vi "Fetch Waveforms for One Record.vi"(8 "error in (no error)":errorcluster, 9 "min record length":i32[](array[numeric]), 10 "fetch record number":i32, 11 "connections":T1[](array[typedef])) -> (0 "error out":errorcluster, 1 "waveforms":waveform(dbl)[](array[waveform]), 2 "sites":i32[](array[numeric]), 3 "pins or relay names":string[](array[string]))   [LabVIEW 2021, in "PMIC Common.lvlib"]
uses:
  PMIC Common.lvlib
  <instrlib>/niScope/Controls/niScope timestamp type.ctl
  <instrlib>/niScope/Acquire/Fetch/niScope Multi Fetch WDT.vi
  <vilib>/Plug-In SDKs/Clients/Session Management V1/Session Reservation/Connection.ctl
  <vilib>/Plug-In SDKs/Clients/Session Management V1/Session Reservation/Session Reservation.lvclass
  <vilib>/Plug-In SDKs/Sessions/niScope/Connection with Session.ctl
  <vilib>/Plug-In SDKs/Sessions/niScope/NI Session Management niScope.lvlib
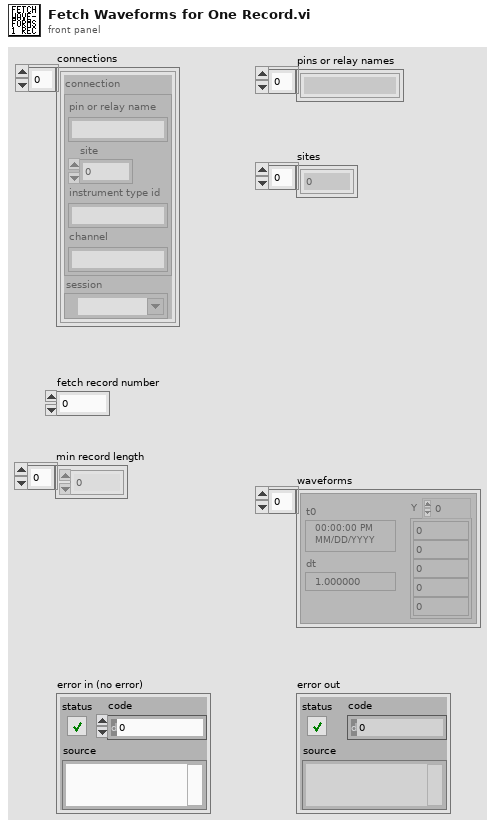
[diagram p1: front panel]
types:
  T1 = typedef "NI Session Management niScope.lvlib/Connection with Session.ctl" = cluster{"connection":T2, "session":refnum<k15>}
  T2 = typedef "NI Session Management V1 Client.lvlib/Session Reservation.lvclass/Connection.ctl" = cluster{"pin or relay name":string, "site":i32, "instrument type id":string, "channel":string}
  T3 = typedef "niScope timestamp type.ctl" = i32
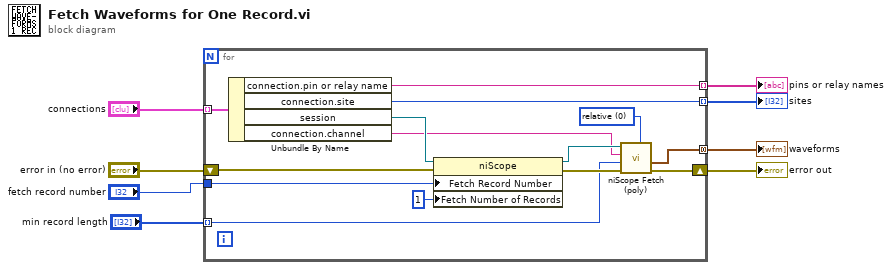
[diagram p0: block diagram]
diagram:
  n1 = for {
    tunnel: "connections" -> [w22] mode=indexing
    tunnel: "fetch record number" -> [w20]
    shift-right: [w14] -> w1
    shift-left: "error in (no error)" -> [w21]
    tunnel: [w13] -> w2 mode=concatenating
    tunnel: "min record length" -> [w12] mode=indexing
    tunnel: [w11] -> w3 mode=indexing
    tunnel: [w10] -> w4 mode=indexing
    w9 = T3 0 items=["relative", "absolute"] ("timestamp Type")
    n2 = Unbundle By Name(w22) -> ("connection.pin or relay name"=w11:string, "connection.site"=w10:i32, "session"=w16:refnum<k15>, "connection.channel"=w15:string)
    n3 = property class="niScope"(reference=w16, error in=w21, "Fetch Record Number"=w20, "Fetch Number of Records"=1 ("Fetch:Fetch Number of Records")) -> (reference out=w17:refnum<k15>, error out=w18:errorcluster)
    n4 = call-poly <instrlib>:"niScope Fetch (poly).vi"("timestamp Type"=w9, "error in"=w18, "numSamples"=w12, "channels"=w15, "instrument handle"=w17) -> ("error out"=w14:errorcluster, "wfm"=w13:waveform(dbl)[])  [unwired: 3 in, 2 out]
  }
  "sites" <- w4
  "pins or relay names" <- w3
  "waveforms" <- w2
  "error out" <- w1
